vi "Extract command.vi"(8 "error in (no error)":errorcluster, 10 "Multipart Msg in":string[](array[string])) -> (0 "error out":errorcluster, 2 "Response":string[](array[string]))   [LabVIEW 2019, in "Service.lvlib"]
uses:
  Service/Service.lvlib
  TypeDefs/set_tx_freq.ctl
  mmW_commands.lvlib
  <vilib>/addons/_JKI.lib/Serialization/JSON/JKI JSON Serialization.lvlib
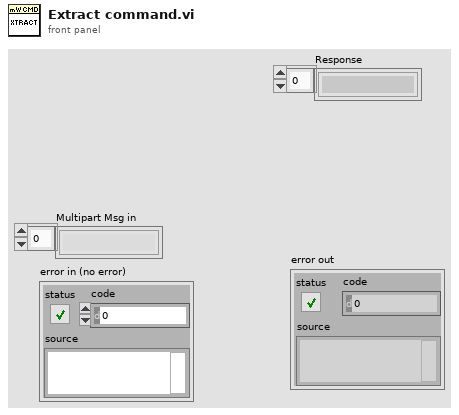
[diagram p1: front panel]
types:
  T1 = typedef "mmW_commands.lvlib/set_tx_freq.ctl" = cluster{"unit":string}
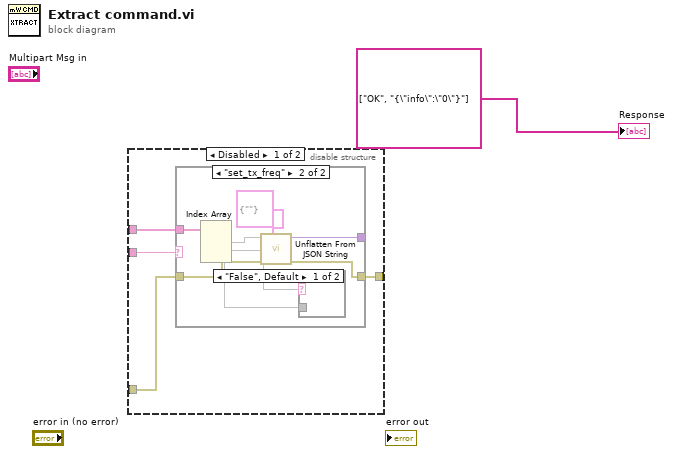
[diagram p0: block diagram]
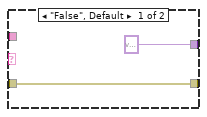
[diagram p2: hidden frame]
diagram:
  n1 = disable-structure shown="Disabled" {
    disable-tunnel: _ -> [w6 _]
    disable-tunnel: _ -> [w4 _]
    disable-tunnel: _ -> [w3 _]
    disable-tunnel: [w2 _] -> _
    frame Disabled {
      n2 = case shown="\"set_tx_freq\"" w4 {
        tunnel: w6 -> [_ w16]
        tunnel: [variant ("Variant") w13] -> w5
        tunnel: w3 -> [w7 w10]
        tunnel: [w7 w9] -> w2
        frame "False", Default {
        }
        frame "set_tx_freq" {
          n3 = Index Array(array=w16) -> (element #1=w15, element #2=w12, element #3=w11)  [unwired: 3 in]
          n4 = call <vilib>:"Unflatten From JSON String.vi"("Type and Defaults"=T1 {"unit"=""}, "error in (no error)"=w10, "JSON String"=w15) -> ("error out"=w9:errorcluster, "Variant"=w13:variant)  [unwired: 7 in]
          n5 = case shown="\"False\", Default" w12 {
            tunnel: w11 -> [_ _]
            frame "False", Default {
            }
            frame "float" {
            }
          }
        }
      }
    }
    frame Enabled {
    }
  }
  "Response" <- string[] ["OK", "{\"info\":\"0\"}"] ("Array")
